vi "Define Default Prefix.vi"(8 "error in (no error)":errorcluster, 11 "PWM Output Channel in":refnum<class "PWM Output Channel.lvclass">) -> (0 "error out":errorcluster, 3 "PWM Output Channel out":refnum<class "PWM Output Channel.lvclass">)   [LabVIEW 2017, in "Scan Engine Scripting.lvlib" / "PWM Output Channel.lvclass"]
doc: "Assigns the default prefix to the channel."
uses:
  PWM Output Channel.lvclass
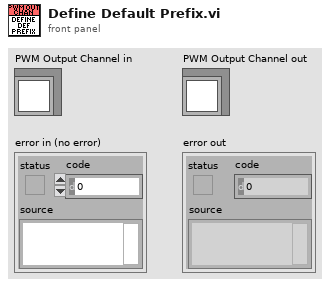
[diagram p1: front panel]
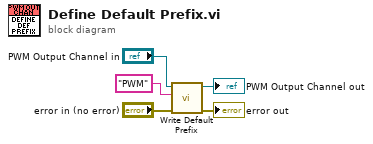
[diagram p0: block diagram]
diagram:
  n1 = call-dynamic "Write Default Prefix.vi"("error in"="error in (no error)", "default prefix"="PWM", "channel in"="PWM Output Channel in") -> ("error out"=→"error out":errorcluster, "channel out"=→"PWM Output Channel out":refnum<class "PWM Output Channel.lvclass">)  [unwired: 7 in]
